vi "Coherent decode tuning.vi"(11 "Tuning string":string) -> (3 "Tuning Desc.":string)   [LabVIEW 2020]
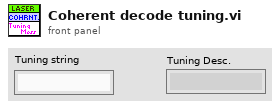
[diagram p1: front panel]
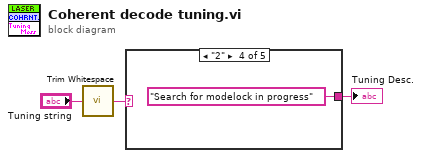
[diagram p0: block diagram]
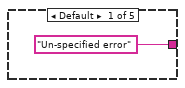
[diagram p2: hidden frame]
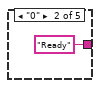
[diagram p3: hidden frame]
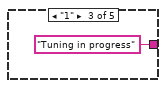
[diagram p4: hidden frame]
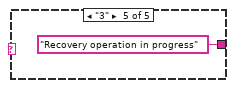
[diagram p5: hidden frame]
diagram:
  n1 = call <vilib>:"Trim Whitespace.vi"("string"="Tuning string") -> ("trimmed string"=w2:string)  [unwired: 1 in]
  n2 = case shown="\"2\"" w2 {
    tunnel: ["Un-specified error" "Ready" "Tuning in progress" "Search for modelock in progress" "Recovery operation in progress"] -> w1
    frame Default {
    }
    frame "0" {
    }
    frame "1" {
    }
    frame "2" {
    }
    frame "3" {
    }
  }
  "Tuning Desc." <- w1
